vi "Test GitHub Issue 51 - Deserialize Array of Cluster with Element of Empty Cluster.vi"(8 "error in":errorcluster) -> (0 "error out":errorcluster)   [LabVIEW 2020]
uses:
  <vilib>/addons/_JKI Toolkits/Caraya/classes/Assert/Assert Equal Value and Type_Variant.vi
  <userlib>/_OpenG.lib/lvdata/lvdata.llb/openg_variant.lvlib
  src/JKI JSON Serialization.lvlib
  <vilib>/addons/_JKI Toolkits/Caraya/classes/Test/Test.lvclass
  <vilib>/addons/_JKI Toolkits/Caraya/classes/Assert/Assert.lvclass
panel:
  out "Array of VData":variant
  out "Variant original":variant
  out "Actual Variant":variant
  in  "jsonText":string="{\n    \"array\": [\n        {\n            \"cluster\": {\n                \"empty_cluster\": {}\n            },\n            \"scalar\": 0\n        }\n    ]\n}"
  in  "approximate jsonText that works":string="\n        {\n            \"cluster\": {\n                \"empty_cluster\": {}\n            },\n            \"scalar\": 0\n        }\n"
  out "Massaged Expected Variant":variant
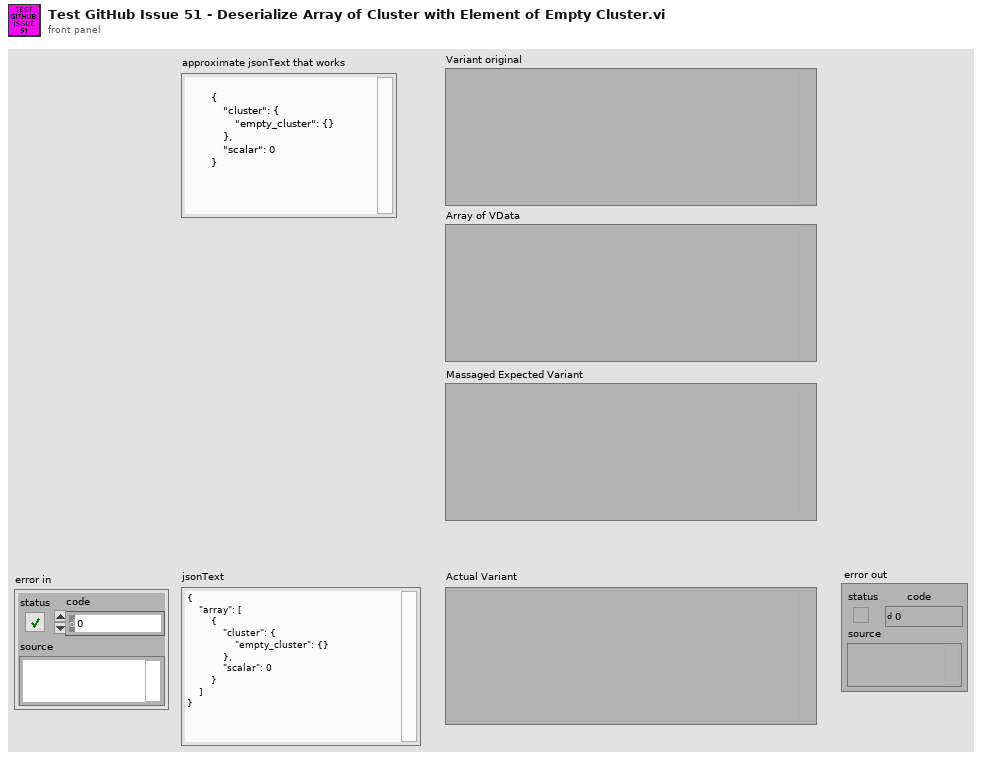
[diagram p1: front panel]
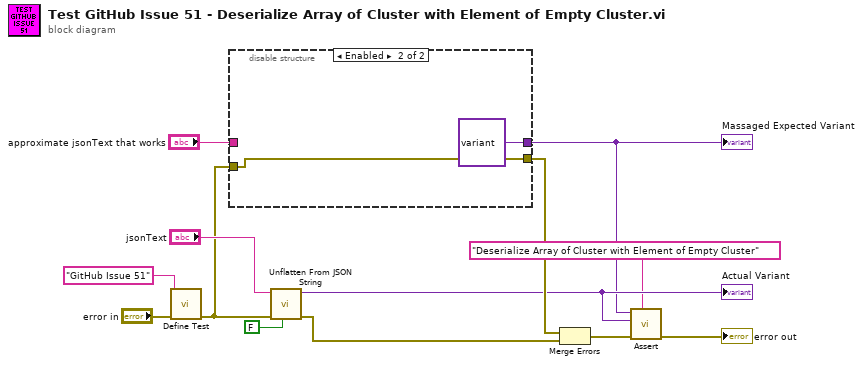
[diagram p0: block diagram]
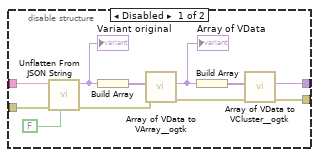
[diagram p2: hidden frame]
diagram:
  n1 = call <vilib>:"Define Test.vi"("error in (no error)"="error in", "Label (VI Title)"="GitHub Issue 51") -> ("error out"=w7:errorcluster)  [unwired: 8 in, 1 out]
  n2 = disable-structure "Diagram Disable Structure" shown="Enabled" {
    disable-tunnel: "approximate jsonText that works" -> [w23 _]
    disable-tunnel: w7 -> [w16 w26]
    disable-tunnel: [w15 w26] -> w6
    disable-tunnel: [w14 variant(cluster{cluster{"cluster":cluster{"empty_cluster":cluster{}}, "scalar":u64}[]} {[{"cluster"={"empty_cluster"={}}, "scalar"=0}]}) ("Massaged Expected Variant")] -> w1
    frame Disabled {
      n3 = call "Unflatten From JSON String.vi"("Nulls as Defaults (F)"=FALSE, "error in"=w16, "JSON String"=w23) -> ("error out"=w21:errorcluster, "Variant"=w18:variant)  [unwired: 7 in]
      "Variant original" <- w18
      n4 = Build Array(w18) -> (w24:variant[])
      n5 = call <userlib>:"Array of VData to VArray__ogtk.vi"("error in (no error)"=w21, "1D Array of VData"=w24) -> ("error out"=w19:errorcluster, "VArray"=w17:variant)  [unwired: 8 in]
      "Array of VData" <- w17
      n6 = Build Array(w17) -> (w20:variant[])
      n7 = call <userlib>:"Array of VData to VCluster__ogtk.vi"("error in (no error)"=w19, "Array"=w20) -> ("error out"=w15:errorcluster, "VCluster"=w14:variant)  [unwired: 8 in]
    }
    frame Enabled {
    }
  }
  "Massaged Expected Variant" <- w1
  n8 = call "Unflatten From JSON String.vi"("Nulls as Defaults (F)"=FALSE, "error in"=w7, "JSON String"="jsonText") -> ("error out"=w12:errorcluster, "Variant"=w4:variant)  [unwired: 7 in]
  "Actual Variant" <- w4
  n9 = Merge Errors(w6, w12) -> (w5:errorcluster)
  n10 = call-poly <vilib>:"Assert.vi"("Label"="Deserialize Array of Cluster with Element of Empty Cluster", "error in (no error)"=w5, "Y"=w4, "X"=w1) -> ("error out"=→"error out":errorcluster)  [unwired: 6 in, 1 out]
